vi "Sensor data.vi"(9 "Update channels":bool, 10 "Sensor Array":T2, 11 "Connection ID in":refnum<k5>) -> (0 "Data Status":T1, 1 "time (s)":dbl format="%.2f", 2 "voltage data":sgl[](array[numeric]) format="%.5f", 3 "Sensor Data":T4 {"Sensor array"."scaled" format="%.2f"; "Sensor array"."voltage" format="%.4f"; "Time" format="%<%I:%M:%S%2u %p\n%m/%d/%Y>T"}, 4 "Data Failure":bool, 5 "Sensor Array out":T2, 6 "error out":errorcluster, 8 "sensor range error":bool)   [LabVIEW 2012]
doc: "Collects one scan of sensor data from the Data Server, scales the data according to scaling selected in the Sensor Array and bundles the data into the Sensor Data cluster.\nSensor Data uses Server Stats to determine if any of the data is at the minimum or maximum for the channel and if so sets the Out of Range indicator to true."
uses:
  Sensor data.ctl
  DAQ configuration/sensor cluster.ctl
  DAQ configuration/Sensor array.ctl
  DAQ configuration/channel identifier.ctl
  Process Controller 3.0/data status.ctl
  Send 1 Scan multi-channel.vi
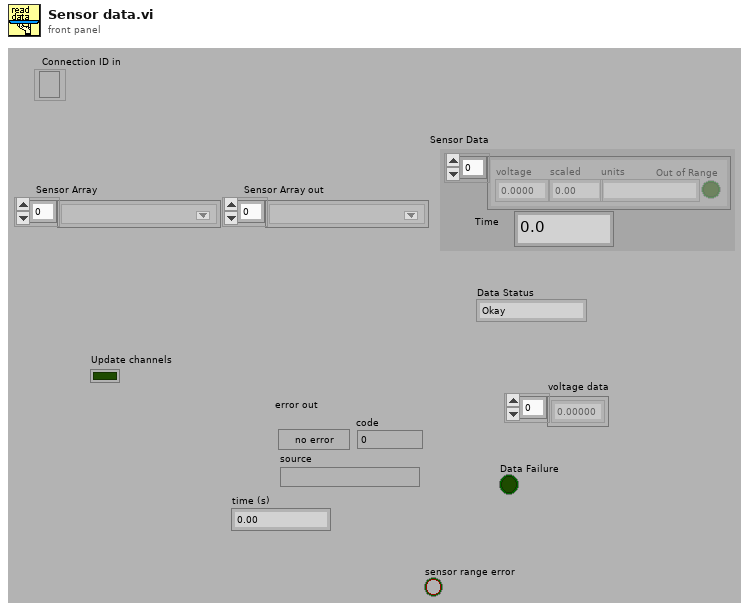
[diagram p1: front panel]
types:
  T1 = typedef "data status.ctl" = enum16{"Okay", "Sensor Range error", "Server error"}
  T2 = typedef "Sensor array.ctl" = T3[]
  T3 = typedef "channel identifier.ctl" = u16
  T4 = typedef "Sensor data.ctl" = cluster{" Sensor array":T5[], "Time":dbl}
  T5 = typedef "sensor cluster.ctl" = cluster{"voltage":sgl, "scaled":sgl, "units":string, "Out of Range":bool}
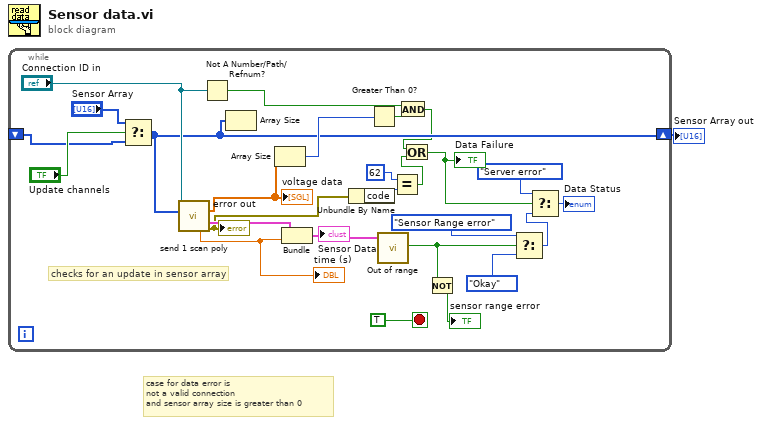
[diagram p0: block diagram]
diagram:
  # "case for data error is\nnot a valid connection\nand sensor array size is greater than 0"
  n1 = while {
    shift-right: [w9] -> w1
    shift-left: _ -> [w13]
    stop <- TRUE stop-if-true
    # "checks for an update in sensor array"
    n2 = Select(t="Sensor Array", s="Update channels", f=w13) -> (s? t:f=w9:T2)
    n3 = call-poly "send 1 scan poly.vi"("Connection ID in"="Connection ID in", "Channel"=w9) -> ("voltage data"=w24:sgl[], "Sensor cluster"=w27:T5[], "time (s)"=w26:dbl, "error out"=w7:errorcluster)  [unwired: 6 in, 4 out]
    "error out" <- w7
    "voltage data" <- w24
    "time (s)" <- w26
    n4 = Not A Number/Path/Refnum?(number/path/refnum="Connection ID in") -> (NaN/Path/Refnum?=w8:bool)
    n5 = Array Size(array=w9) -> ()  [unwired: 1 out]
    n6 = Array Size(array=w24) -> (size(s)=w10:i32)
    n7 = Bundle("Sensor cluster"=w27, "time (s)"=w26) -> (w23:cluster{"Sensor cluster":T5[], "time (s)":dbl})  [unwired: 1 in]
    "Sensor Data" <- w23
    n8 = Unbundle By Name(w7) -> ("code"=w5:i32)
    n9 = Greater Than 0?(x=w10) -> (x > 0?=w11:bool)
    n10 = call "Out of range.vi"("Sensor Data"=w23) -> ("Out of Range"=w17:bool)  [unwired: 6 in]
    n11 = Equal?(x=62, y=w5) -> (x = y?=w3:bool)
    n12 = And(x=w8, y=w11) -> (x .and. y?=w4:bool)
    n13 = Or(x=w4, y=w3) -> (x .or. y?=w2:bool)
    "Data Failure" <- w2
    n14 = Not(x=w17) -> (.not. x?=→"sensor range error":bool)
    n15 = Select(t=data_status."Sensor Range error" ("Data Status"), s=w17, f=data_status."Okay" ("Data Status")) -> (s? t:f=w21:T1)
    n16 = Select(t=data_status."Server error" ("Data Status"), s=w2, f=w21) -> (s? t:f=→"Data Status":T1)
  }
  "Sensor Array out" <- w1
